vi "Persist Config.vi"(7 "Name Delimiter":string, 8 "error in (no error)":errorcluster, 10 "Elements":refnum<class "Config Element.lvclass">[](array[class]), 11 "Config-Sqlite in":refnum<class "Config-Sqlite.lvclass">) -> (0 "error out":errorcluster, 3 "Config-Sqlite out":refnum<class "Config-Sqlite.lvclass">)   [LabVIEW 2020, in "CDM-Config.lvlib" / "Config-Sqlite.lvclass"]
uses:
  Config-Sqlite.lvclass
  Config Element/Config Element.lvclass
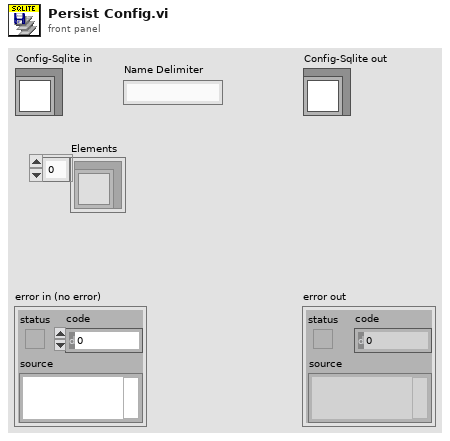
[diagram p1: front panel]
types:
  T1 = cluster{i32, "Element Ref":refnum<class "Config Element.lvclass">}
  T2 = cluster{"Row":i32, "Elements":refnum<class "Config Element.lvclass">}
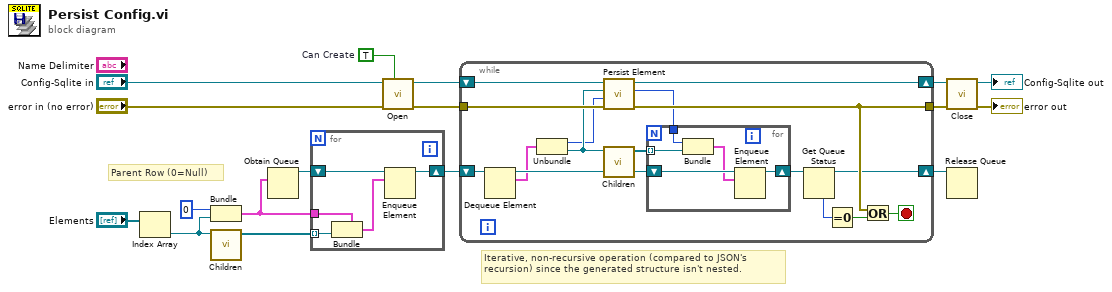
[diagram p0: block diagram]
diagram:
  w1 = TRUE  # Can Create
  # "Iterative, non-recursive operation (compared to JSON's recursion) since the generated structure isn't nested."
  # "Parent Row (0=Null)"
  n1 = Index Array(array="Elements") -> (element=w3:refnum<class "Config Element.lvclass">)  [unwired: 1 in]
  n2 = Bundle(0, "Element Ref"=w3) -> (w4:T1)  [unwired: 1 in]
  n3 = call "Children.vi"("Config Element in"=w3) -> ("Elements"=w2:refnum<class "Config Element.lvclass">[])  [unwired: 9 in, 1 out]
  n4 = Obtain Queue(element data type=w4) -> (queue out=w14:refnum<queue>)  [unwired: 4 in, 2 out]
  n5 = for {
    shift-right: [w21] -> w11
    shift-left: w14 -> [w22]
    tunnel: w4 -> [w20]
    tunnel: w2 -> [w19] mode=indexing
    n6 = Bundle(cluster=w20, "Element Ref"=w19) -> (w18:T1)  [unwired: 1 in]
    n7 = Enqueue Element(queue=w22, element=w18) -> (queue out=w21:refnum<queue>)  [unwired: 2 in, 2 out]
  }
  n8 = call "Open.vi"("Can Create"=w1, "error in (no error)"="error in (no error)", "Config-Sqlite in"="Config-Sqlite in") -> ("error out"=w12:errorcluster, "Config-Sqlite out"=w13:refnum<class "Config-Sqlite.lvclass">)  [unwired: 7 in]
  n9 = while {
    shift-right: [w27] -> w8
    shift-left: w13 -> [w33]
    tunnel: w12 -> [w32]
    shift-right: [w36] -> w5
    shift-left: w11 -> [w37]
    tunnel: [w38] -> w10
    stop <- w26 stop-if-true
    n10 = Dequeue Element(queue=w37) -> (queue out=w31:refnum<queue>, element=w29:T1)  [unwired: 2 in, 2 out]
    n11 = Unbundle(w29) -> (w23:i32, "Element Ref"=w24:refnum<class "Config Element.lvclass">)
    n12 = call "Persist Element.vi"("error in (no error)"=w32, "Parent"=w23, "Element"=w24, "Config-Sqlite in"=w33) -> ("error out"=w38:errorcluster, "Row"=w25:i32, "Config-Sqlite out"=w27:refnum<class "Config-Sqlite.lvclass">)  [unwired: 5 in]
    n13 = call "Children.vi"("Config Element in"=w24) -> ("Elements"=w30:refnum<class "Config Element.lvclass">[])  [unwired: 9 in, 1 out]
    n14 = for {
      shift-right: [w42] -> w28
      shift-left: w31 -> [w43]
      tunnel: w30 -> [w41] mode=indexing
      tunnel: w25 -> [w40]
      n15 = Bundle("Row"=w40, "Elements"=w41) -> (w39:T2)  [unwired: 1 in]
      n16 = Enqueue Element(queue=w43, element=w39) -> (queue out=w42:refnum<queue>)  [unwired: 2 in, 2 out]
    }
    n17 = Get Queue Status(queue=w28) -> (queue out=w36:refnum<queue>, # elements in queue=w35:i32)  [unwired: 2 in, 6 out]
    n18 = Equal To 0?(x=w35) -> (x = 0?=w34:bool)
    n19 = Or(x=w38, y=w34) -> (x .or. y?=w26:bool)
  }
  n20 = call "Close.vi"("error in (no error)"=w10, "Config-Sqlite in"=w8) -> ("error out"=→"error out":errorcluster, "Config-Sqlite out"=→"Config-Sqlite out":refnum<class "Config-Sqlite.lvclass">)  [unwired: 8 in]
  n21 = Release Queue(queue=w5) -> ()  [unwired: 2 in, 3 out]
